vi "Get egg5302 Formated Parameters VISA.VI"(8 "error in (no error)":errorcluster, 10 "Input String":string, 11 "GPIB Address":i16=6) -> (0 "error out":errorcluster, 1 "Time Constant":dbl format="%.2e", 2 "Sensitivity":dbl format="%.4e", 3 "Frequency":dbl format="%.2e", 4 "Phase":dbl format="%.2f", 5 "Oscillator voltage":dbl format="%.2e", 6 "Parameters":string)   [LabVIEW 2015]
panel:
  in  "VISA session (for class)":refnum<visa-resource-name>
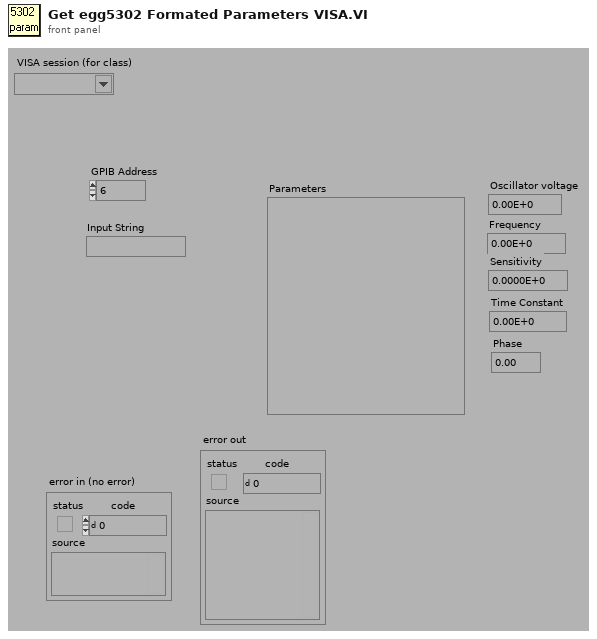
[diagram p1: front panel]
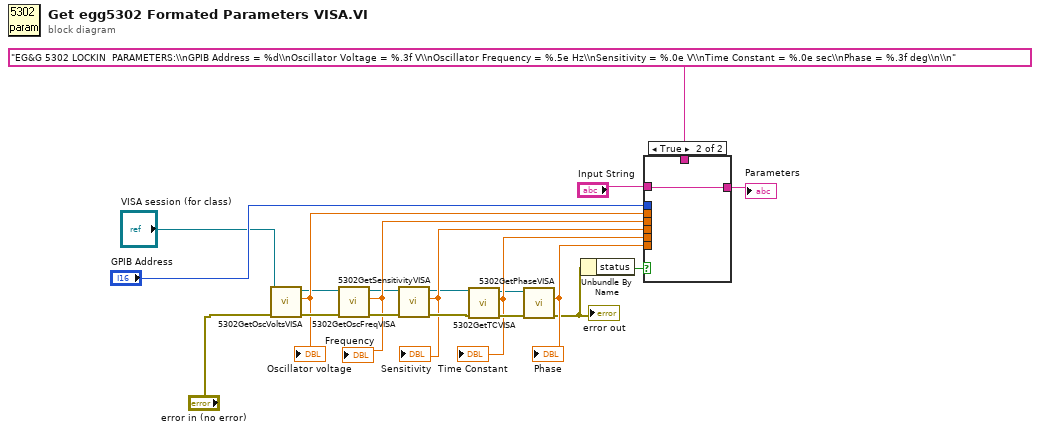
[diagram p0: block diagram]
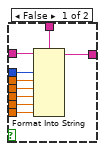
[diagram p2: hidden frame]
diagram:
  n1 = call "5302GetOscVoltsVISA.vi"("error in (no error)"="error in (no error)", "VISA session (for class)"="VISA session (for class)") -> ("error out"=w21:errorcluster, "Osc Volts"=w13:dbl, "VISA session"=w5:refnum<visa-resource-name>)  [unwired: 6 in, 1 out]
  "Oscillator voltage" <- w13
  n2 = call "5302GetOscFreqVISA.vi"("error in (no error)"=w21, "VISA session (for class)"=w5) -> ("error out"=w20:errorcluster, "Osc Freq"=w14:dbl, "VISA session"=w4:refnum<visa-resource-name>)  [unwired: 6 in, 1 out]
  "Frequency" <- w14
  n3 = call "5302GetSensitivityVISA.vi"("error in (no error)"=w20, "VISA session (for class)"=w4) -> ("error out"=w19:errorcluster, "Sevsitivity"=w15:dbl, "VISA session"=w2:refnum<visa-resource-name>)  [unwired: 6 in, 1 out]
  "Sensitivity" <- w15
  n4 = call "5302GetTCVISA.vi"("error in (no error)"=w19, "VISA session (for class)"=w2) -> ("error out"=w18:errorcluster, "Time Constant"=w16:dbl, "VISA session"=w1:refnum<visa-resource-name>)  [unwired: 6 in, 1 out]
  "Time Constant" <- w16
  n5 = call "5302GetPhaseVISA.vi"("error in (no error)"=w18, "VISA session (for class)"=w1) -> ("error out"=w11:errorcluster, "Phase"=w17:dbl)  [unwired: 6 in, 2 out]
  "error out" <- w11
  "Phase" <- w17
  n6 = Unbundle By Name(w11) -> ("status"=w10:bool)
  n7 = case shown="True" w10 {
    tunnel: w17 -> [w30 _]
    tunnel: w16 -> [w29 _]
    tunnel: w15 -> [w28 _]
    tunnel: w14 -> [w27 _]
    tunnel: w13 -> [w26 _]
    tunnel: "GPIB Address" -> [w25 _]
    tunnel: "EG&G 5302 LOCKIN  PARAMETERS:\\nGPIB Address = %d\\nOscillator Voltage = %.3f V\\nOscillator Frequency = %.5e Hz\\nSensitivity = %.0e V\\nTime Constant = %.0e sec\\nPhase = %.3f deg\\n\\n" -> [w24 _]
    tunnel: "Input String" -> [w23 w31]
    tunnel: [w22 w31] -> w8
    frame False {
      n8 = Format Into String(format string=w24, initial string=w23, w25, w26, w27, w28, w29, w30) -> (resulting string=w22:string)  [unwired: 1 in, 1 out]
    }
    frame True {
    }
  }
  "Parameters" <- w8
